vi "unique-name-multiple-instances.vi"(8 "error in (no error)":errorcluster) -> (0 "error out":errorcluster)   [LabVIEW 2021]
uses:
  <vilib>/addons/_JKI Toolkits/Caraya/classes/Test/Test.lvclass
  src/SMO/SMO.lvclass
  <vilib>/addons/_JKI Toolkits/Caraya/classes/Assert/Assert.lvclass
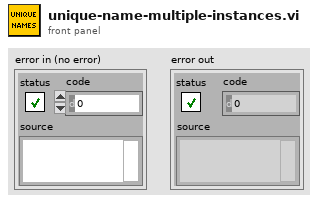
[diagram p1: front panel]
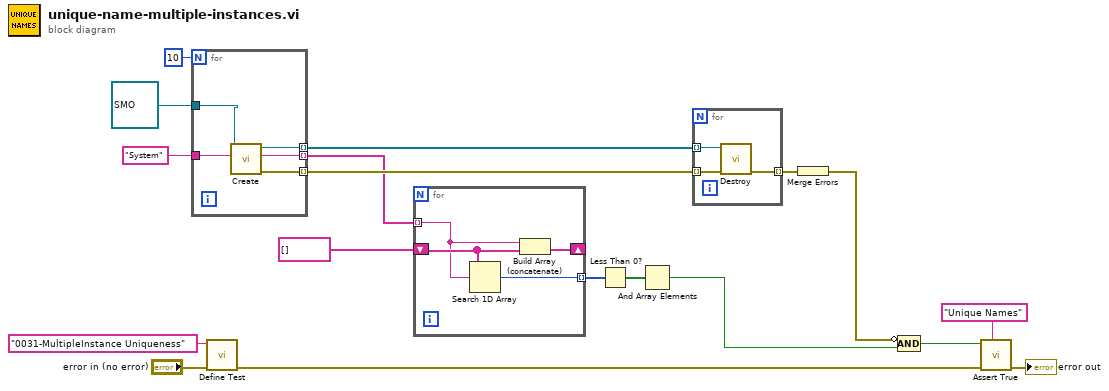
[diagram p0: block diagram]
diagram:
  n1 = for {
    N: 10 -> [_]
    tunnel: "System" ("Subsystem Name (optional)") -> [w23]
    tunnel: [w22] -> w5 mode=indexing
    tunnel: [w21] -> w11 mode=indexing
    tunnel: [w20] -> w8 mode=indexing
    tunnel: refnum<class "SMO.lvclass"> refnum ("Dependency Type") -> [w19]
    n2 = call "Create.vi"("Subsystem Name (optional)"=w23, "SMO"=w19) -> ("error out"=w20:errorcluster, "SMO name"=w22:string, "SMO out"=w21:refnum<class "SMO.lvclass">)  [unwired: 7 in]
  }
  n3 = call <vilib>:"Define Test.vi"("error in (no error)"="error in (no error)", "Label (VI Title)"="0031-MultipleInstance Uniqueness") -> ("error out"=w7:errorcluster)  [unwired: 9 in]
  n4 = for {
    shift-right: [w25] -> _
    shift-left: string[] [] -> [w27]
    tunnel: w5 -> [w26] mode=indexing
    tunnel: [w24] -> w4 mode=indexing
    n5 = Search 1D Array(1D array=w27, element=w26) -> (index of element=w24:i32)  [unwired: 1 in]
    n6 = Build Array (concatenate)(w26, w27) -> (w25:string[])
  }
  n7 = Less Than 0?(x=w4) -> (x < 0?=w3:bool[])
  n8 = And Array Elements(Boolean array=w3) -> (logical AND=w2:bool)
  n9 = for {
    tunnel: w11 -> [w30] mode=indexing
    tunnel: [w29] -> w10 mode=indexing
    tunnel: w8 -> [w28] mode=indexing
    n10 = call "Destroy.vi"("error in (no error)"=w28, "SMO"=w30) -> ("error out"=w29:errorcluster)  [unwired: 9 in]
  }
  n11 = Merge Errors(w10) -> (w9:errorcluster)
  n12 = Compound Arithmetic op=AND(invert w9, w2) -> (w14:bool)
  n13 = call <vilib>:"Assert True.vi"("Label"="Unique Names" ("Label (VI Title)"), "error in (no error)"=w7, "True?"=w14) -> ("error out"=→"error out":errorcluster)  [unwired: 8 in]
